vi "Write to TCP.vi"(8 "error in (no error)":errorcluster, 11 "Vessel in":refnum<class "Vessel.lvclass">) -> (0 "error out":errorcluster, 3 "Vessel out":refnum<class "Vessel.lvclass">)   [LabVIEW 2014, in "Vessel.lvclass"]
uses:
  Vessel.lvclass
  Vessel.lvclass/Vessel.ctl
  Library/Helping Routines/get_set_point (SubVI).vi
  Supervisor/Supervisor.lvclass
panel:
  out "Name":string
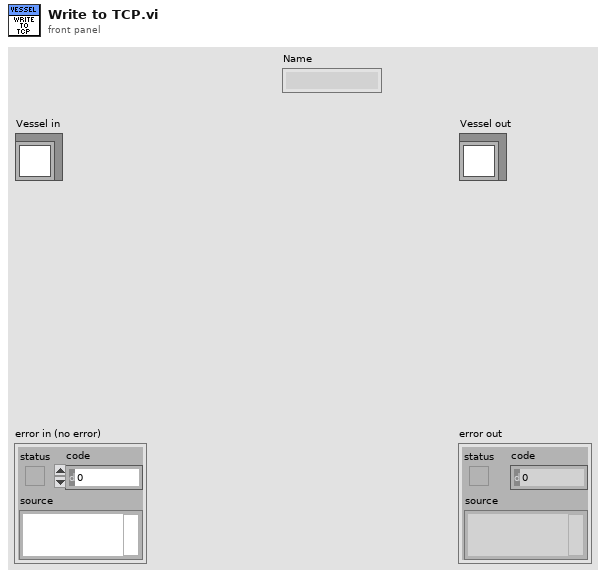
[diagram p1: front panel]
types:
  T1 = cluster{"Measured":cluster{"Eta":dbl[], "Nu":dbl[], "Eta Dot":dbl[], "Nu Dot":dbl[]}, "Estimated":cluster{"Eta":dbl[], "Nu":dbl[], "Eta Dot":dbl[], "Nu Dot":dbl[]}, "Desired":cluster{"Eta":dbl[], "Nu":dbl[], "Eta Dot":dbl[], "Nu Dot":dbl[]}, "Previous Desired":cluster{"Eta":dbl[], "Nu":dbl[], "Eta Dot":dbl[], "Nu Dot":dbl[]}, "tau":dbl[], "Altitude":cluster{"Measured":dbl, "Estimated":dbl, "Desired":dbl, "Previous Desired":dbl, "Approximated":dbl, "grad F":dbl[]}, "rpm":dbl[], "Attitude":cluster{"Theta Measured":dbl[], "Theta Estimated":dbl[], "Omega Measured":dbl[], "Omega Estimated":dbl[], "Gyro Bias":dbl[]}}
  T2 = cluster{"Set Origin":bool, "New WP":bool, "Types of Change":enum16{"Current NED", "Change NED"}, "Make Change":bool, "Optimal Heading":bool, "New SetPoint":cluster{"North":dbl, "East":dbl, "Depth":dbl, "Heading":dbl}, "Update Reference":cluster{"Mode Change":bool, "Current Position":dbl[]}, "Go":bool, "Go heading":bool}
  T3 = cluster{"Pressure +":bool, "Pressure -":bool, "Vacuum +":bool, "Vacuum -":bool}
  T4 = cluster{"In":bool, "Out":bool, "Rotate CW":bool, "Rotate CCW":bool}
  T5 = cluster{"Button 1":bool, "Button 2":bool, "Button 3":bool, "Button 4":bool, "Button 5":bool, "Button 6":bool, "Button 7":bool, "Button 8":bool, "Button 9":bool, "Button 10":bool, "Button 11":bool, "Button 12":bool, "POV Direction":i32}
  T6 = cluster{"Eta":dbl[], "Nu":dbl[], "Eta Dot":dbl[], "Nu Dot":dbl[]}
  T7 = cluster{"Theta Measured":dbl[], "Theta Estimated":dbl[], "Omega Measured":dbl[], "Omega Estimated":dbl[], "Gyro Bias":dbl[]}
  T8 = cluster{"Measured":dbl, "Estimated":dbl, "Desired":dbl, "Previous Desired":dbl, "Approximated":dbl, "grad F":dbl[]}
  T9 = cluster{"HPR":bool, "Sonar 1":bool, "Sonar 2":bool, "Doppler":bool, "Laser":bool, "KRAFT":bool, "Pan/Tilt":bool, "Transponder":bool, "Still Cam":bool, "HD Cam":bool, "UHI Cam":bool}
  T10 = cluster{"Power Switch":bool, "Upper Arm Up":bool, "Upper Arm Down":bool, "Lower Arm Up":bool, "Lower Arm Down":bool, "Arm Left":bool, "Arm Right":bool, "Claw Open":bool, "Claw Close":bool, "Rotate Clockwise":bool, "Rotate Counterclockwise":bool}
  T11 = cluster{"Light 1":bool, "Light 2":bool, "Light 3":bool, "Light 4":bool, "HMI 1":bool, "HMI 2":bool, "Light Intensity 1":i32, "Light Intensity 2":i32, "Light Intensity 3":i8}
  T12 = cluster{"Cam. No.":i32, "Cam Up":bool, "Cam Down":bool, "Cam Left":bool, "Cam Right":bool, "Zoom In":bool, "Zoom Out":bool, "Zoom In 2":bool, "Zoom Out 2":bool}
  T13 = cluster{"Altimeter Active":bool, "Beam select":i8, "Value":cluster{"Measured":dbl, "Estimated":dbl, "Desired":dbl, "Previous Desired":dbl, "Approximated":dbl}}
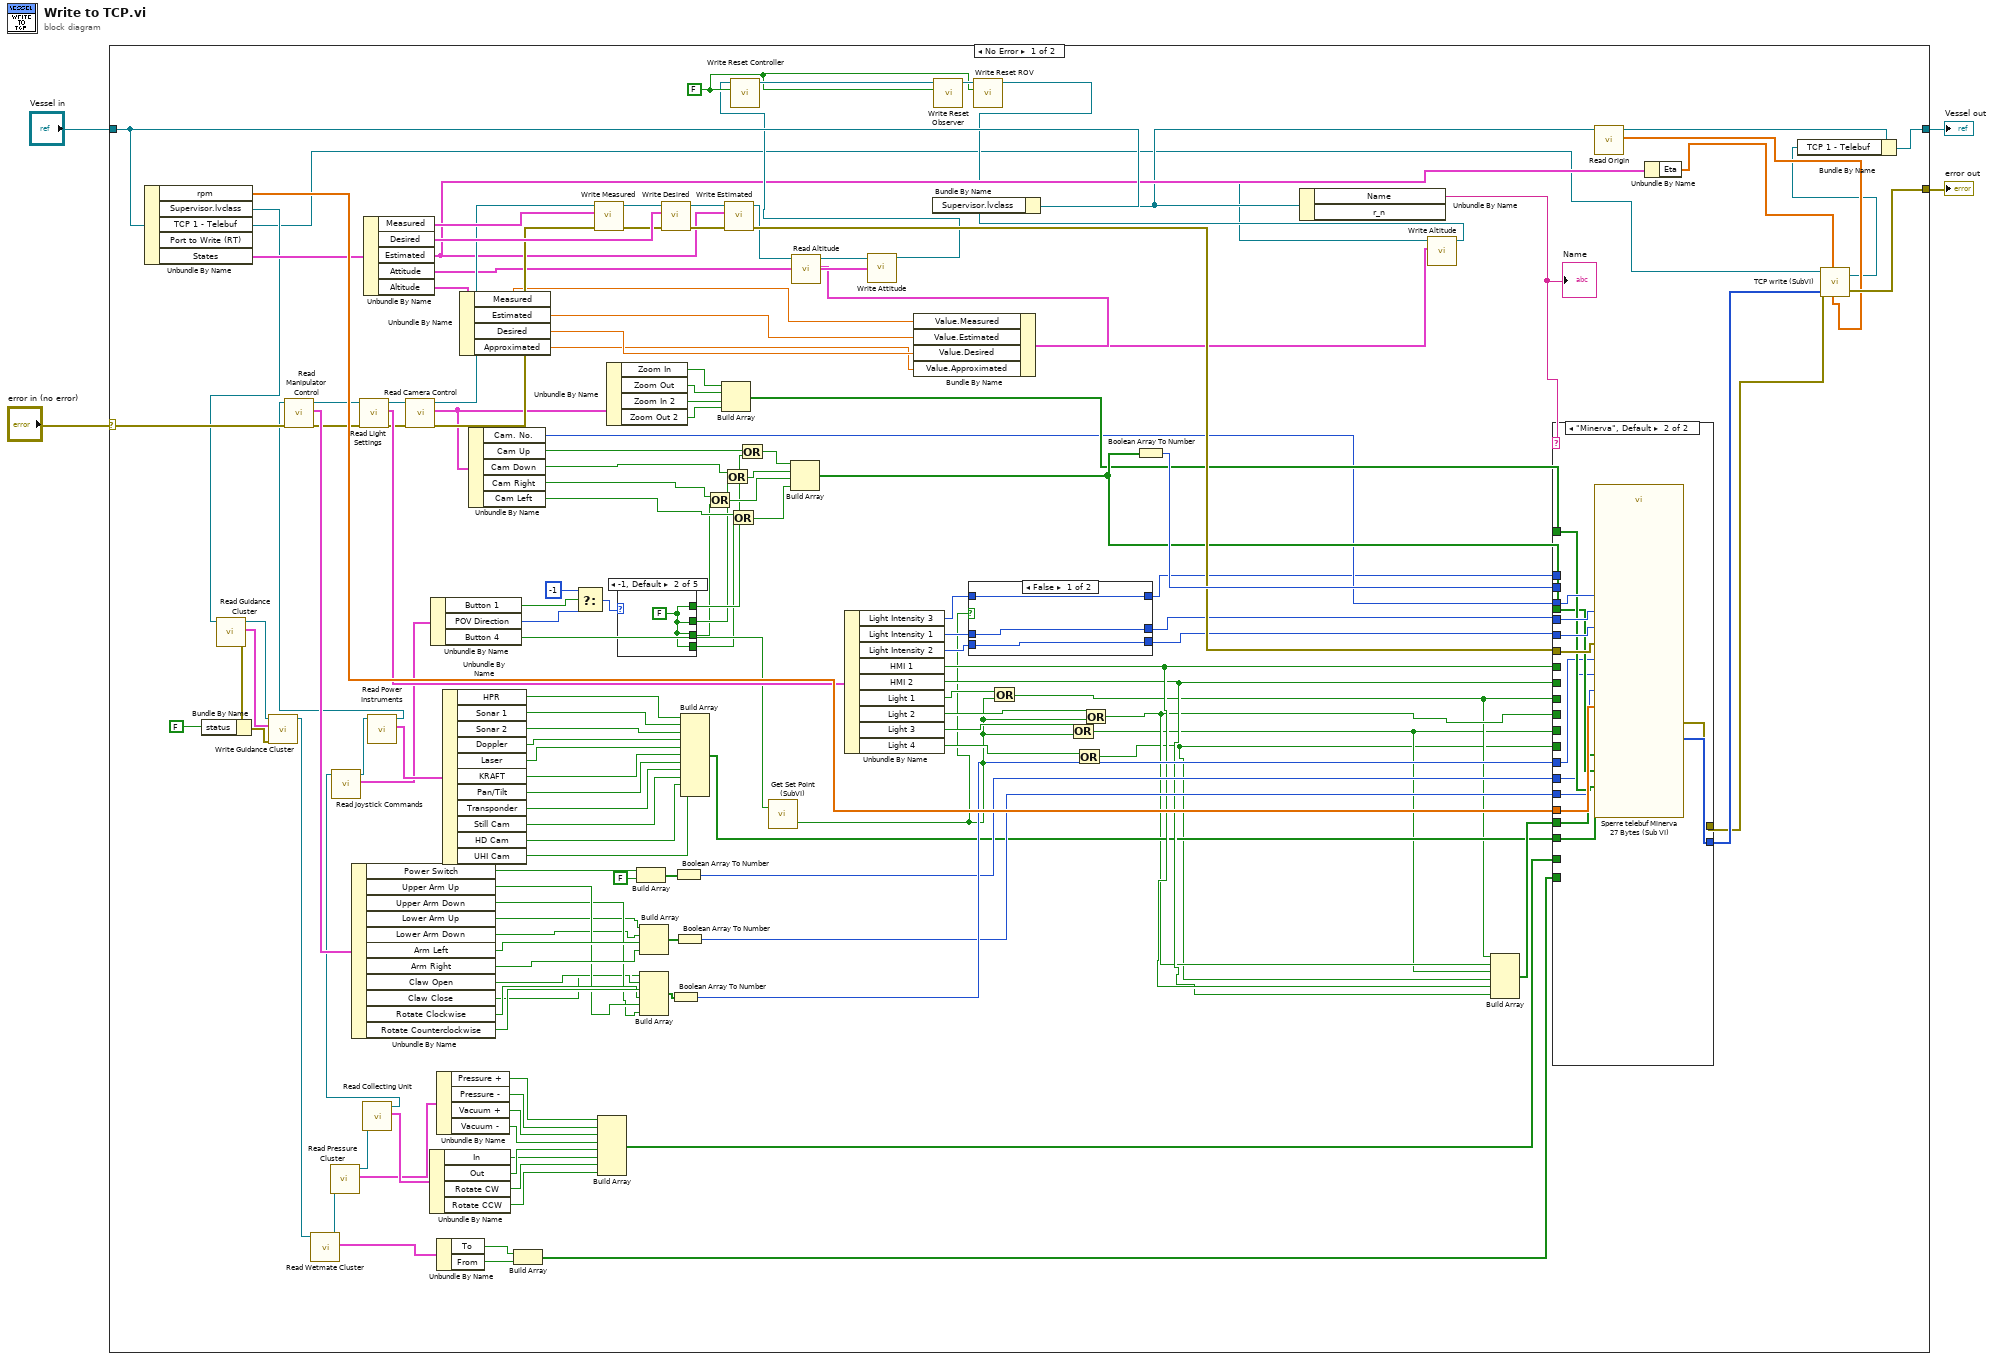
[diagram p0: block diagram]
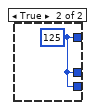
[diagram p2: hidden frame]
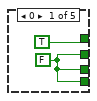
[diagram p3: hidden frame]
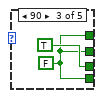
[diagram p4: hidden frame]
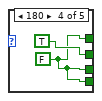
[diagram p5: hidden frame]
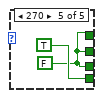
[diagram p6: hidden frame]
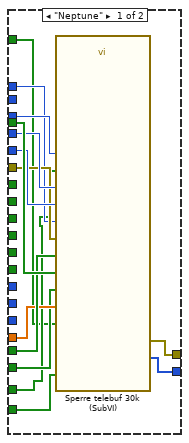
[diagram p7: hidden frame]
diagram:
  n1 = case shown="No Error" "error in (no error)" {
    selector: "error in (no error)" -> [w141 w197]
    tunnel: [w9 w197] -> w3
    tunnel: [w144 w196] -> w1
    tunnel: "Vessel in" -> [w133 w196]
    frame No Error {
      w121 = FALSE ("Reset Controller")
      n2 = Unbundle By Name(w133) -> ("rpm"=w154:dbl[], "Supervisor.lvclass"=w124:refnum<class "Supervisor.lvclass">, "TCP 1 - Telebuf"=w6:refnum<k5>, "States"=w138:T1)  [unwired: 1 out]
      n3 = call-dynamic "Read Guidance Cluster.vi"("Supervisor in"=w124) -> ("error out"=w126:errorcluster, "Guidance Cluster"=w65:T2, "Supervisor out"=w127:refnum<class "Supervisor.lvclass">)  [unwired: 8 in]
      n4 = Bundle By Name(cluster=w126, "status"=FALSE ("Set Origin")) -> (w66:errorcluster)
      n5 = call-dynamic "Write Guidance Cluster.vi"("error in (no error)"=w66, "Guidance Cluster"=w65, "Supervisor in"=w127) -> ("Supervisor out"=w73:refnum<class "Supervisor.lvclass">)  [unwired: 7 in, 1 out]
      n6 = call-dynamic "Read Wetmate Cluster.vi"("Supervisor in"=w73) -> ("Wetmate Cluster"=w71:cluster{"To":bool, "From":bool}, "Supervisor out"=w72:refnum<class "Supervisor.lvclass">)  [unwired: 8 in, 1 out]
      n7 = call-dynamic "Read Pressure Cluster.vi"("Supervisor in"=w72) -> ("Pressure Cluster"=w78:T3, "Supervisor out"=w79:refnum<class "Supervisor.lvclass">)  [unwired: 8 in, 1 out]
      n8 = call-dynamic "Read Collecting Unit.vi"("Supervisor in"=w79) -> ("Collecting Unit"=w103:T4, "Supervisor out"=w63:refnum<class "Supervisor.lvclass">)  [unwired: 8 in, 1 out]
      n9 = call-dynamic "Read Joystick Commands.vi"("Supervisor in"=w63) -> ("Joystick Commands"=w61:T5, "Supervisor out"=w62:refnum<class "Supervisor.lvclass">)  [unwired: 8 in, 1 out]
      n10 = Unbundle By Name(w138) -> ("Measured"=w137:T6, "Desired"=w136:T6, "Estimated"=w67:T6, "Attitude"=w92:T7, "Altitude"=w85:T8)
      n11 = call-dynamic "Read Power Instruments.vi"("Supervisor in"=w62) -> ("Power Instruments"=w115:T9, "Supervisor out"=w116:refnum<class "Supervisor.lvclass">)  [unwired: 8 in, 1 out]
      n12 = call-dynamic "Read Manipulator Control.vi"("error in (no error)"=w141, "Supervisor in"=w116) -> ("error out"=w140:errorcluster, "Manipulator Control"=w151:T10, "Supervisor out"=w143:refnum<class "Supervisor.lvclass">)  [unwired: 7 in]
      n13 = Unbundle By Name(w151) -> ("Power Switch"=w150:bool, "Upper Arm Up"=w29:bool, "Upper Arm Down"=w28:bool, "Lower Arm Up"=w27:bool, "Lower Arm Down"=w26:bool, "Arm Left"=w34:bool, "Arm Right"=w33:bool, "Claw Open"=w25:bool, "Claw Close"=w24:bool, "Rotate Clockwise"=w30:bool, "Rotate Counterclockwise"=w31:bool)
      n14 = call-dynamic "Read Light Settings.vi"("error in (no error)"=w140, "Supervisor in"=w143) -> ("error out"=w139:errorcluster, "Light Settings"=w152:T11, "Supervisor out"=w142:refnum<class "Supervisor.lvclass">)  [unwired: 7 in]
      n15 = call-dynamic "Read Camera Control.vi"("error in (no error)"=w139, "Supervisor in"=w142) -> ("error out"=w132:errorcluster, "Camera Control"=w97:T12, "Supervisor out"=w134:refnum<class "Supervisor.lvclass">)  [unwired: 7 in]
      n16 = Unbundle By Name(w103) -> ("In"=w101:bool, "Out"=w102:bool, "Rotate CW"=w100:bool, "Rotate CCW"=w99:bool)
      n17 = Unbundle By Name(w61) -> ("Button 1"=w39:bool, "POV Direction"=w38:i32, "Button 4"=w60:bool)
      n18 = Unbundle By Name(w78) -> ("Pressure +"=w77:bool, "Pressure -"=w76:bool, "Vacuum +"=w75:bool, "Vacuum -"=w74:bool)
      n19 = Unbundle By Name(w71) -> ("To"=w70:bool, "From"=w69:bool)
      n20 = Unbundle By Name(w115) -> ("HPR"=w114:bool, "Sonar 1"=w113:bool, "Sonar 2"=w112:bool, "Doppler"=w111:bool, "Laser"=w110:bool, "KRAFT"=w109:bool, "Pan/Tilt"=w108:bool, "Transponder"=w107:bool, "Still Cam"=w106:bool, "HD Cam"=w105:bool, "UHI Cam"=w12:bool)
      n21 = Unbundle By Name(w85) -> ("Measured"=w84:dbl, "Estimated"=w83:dbl, "Desired"=w82:dbl, "Approximated"=w80:dbl)
      n22 = Unbundle By Name(w97) -> ("Cam. No."=w64:i32, "Cam Up"=w51:bool, "Cam Down"=w49:bool, "Cam Right"=w47:bool, "Cam Left"=w45:bool)
      n23 = Build Array(w70, w69) -> (w68:bool[])
      n24 = Select(t=-1, s=w39, f=w38) -> (s? t:f=w37:i32)
      n25 = call-dynamic "Write Measured.vi"("error in (no error)"=w132, "Measured"=w137, "Supervisor in"=w134) -> ("error out"=w131:errorcluster, "Supervisor out"=w135:refnum<class "Supervisor.lvclass">)  [unwired: 7 in]
      n26 = Build Array(w77, w76, w75, w74, w102, w101, w100, w99) -> (w98:bool[])
      n27 = Unbundle By Name(w97) -> ("Zoom In"=w96:bool, "Zoom Out"=w95:bool, "Zoom In 2"=w94:bool, "Zoom Out 2"=w93:bool)
      n28 = case shown="-1, Default" w37 {
        tunnel: [TRUE w161 w162 w164 w166] -> w43
        tunnel: [w159 w161 w162 TRUE w166] -> w42
        tunnel: [w159 w161 TRUE w164 w166] -> w41
        tunnel: [w159 w161 w162 w164 TRUE] -> w40
        frame 0 {
          w159 = FALSE
        }
        frame -1, Default {
          w161 = FALSE
        }
        frame 90 {
          w162 = FALSE
        }
        frame 180 {
          w164 = FALSE
        }
        frame 270 {
          w166 = FALSE
        }
      }
      n29 = Build Array(w150, FALSE ("element")) -> (w149:bool[])
      n30 = Build Array(w27, w26, w34, w33) -> (w32:bool[])
      n31 = Build Array(w24, w25, w31, w30, w29, w28) -> (w148:bool[])
      n32 = call-dynamic "Write Desired.vi"("error in (no error)"=w131, "Desired"=w136, "Supervisor in"=w135) -> ("error out"=w129:errorcluster, "Supervisor out"=w130:refnum<class "Supervisor.lvclass">)  [unwired: 7 in]
      n33 = Boolean Array To Number(Boolean array=w148) -> (number=w147:u32)
      n34 = Boolean Array To Number(Boolean array=w149) -> (number=w146:u32)
      n35 = Boolean Array To Number(Boolean array=w32) -> (number=w145:u32)
      n36 = Build Array(w114, w113, w112, w111, w110, w109, w108, w107, w106, w105, w12) -> (w104:bool[])
      n37 = Or(x=w47, y=w41) -> (x .or. y?=w46:bool)
      n38 = Build Array(w96, w95, w94, w93) -> (w81:bool[])
      n39 = Or(x=w49, y=w42) -> (x .or. y?=w48:bool)
      n40 = call-dynamic "Write Estimated.vi"("error in (no error)"=w129, "Estimated"=w67, "Supervisor in"=w130) -> ("error out"=w128:errorcluster, "Supervisor out"=w89:refnum<class "Supervisor.lvclass">)  [unwired: 7 in]
      n41 = Or(x=w45, y=w40) -> (x .or. y?=w44:bool)
      n42 = Or(x=w51, y=w43) -> (x .or. y?=w50:bool)
      n43 = call-poly "Get Set Point (SubVI).vi"("auto set  in"=w60) -> ("auto set"=w13:bool)  [unwired: 1 in, 1 out]
      n44 = Build Array(w50, w48, w46, w44) -> (w120:bool[])
      n45 = call-dynamic "Read Altitude.vi"("Supervisor in"=w89) -> ("Altitude"=w90:T13, "Supervisor out"=w88:refnum<class "Supervisor.lvclass">)  [unwired: 8 in, 1 out]
      n46 = Unbundle By Name(w152) -> ("Light Intensity 3"=w18:i8, "Light Intensity 1"=w16:i32, "Light Intensity 2"=w14:i32, "HMI 1"=w119:bool, "HMI 2"=w118:bool, "Light 1"=w59:bool, "Light 2"=w58:bool, "Light 3"=w55:bool, "Light 4"=w53:bool)
      n47 = call-dynamic "Write Attitude.vi"("Attitude"=w92, "Supervisor in"=w88) -> ("Supervisor out"=w91:refnum<class "Supervisor.lvclass">)  [unwired: 8 in, 1 out]
      n48 = call-dynamic "Write Reset Controller.vi"("Reset Controller"=w121, "Supervisor in"=w91) -> ("Supervisor out"=w123:refnum<class "Supervisor.lvclass">)  [unwired: 8 in, 1 out]
      n49 = Bundle By Name(cluster=w90, "Value.Measured"=w84, "Value.Estimated"=w83, "Value.Desired"=w82, "Value.Approximated"=w80) -> (w87:T13)
      n50 = call-dynamic "Write Reset Observer.vi"("Reset Observer"=w121, "Supervisor in"=w123) -> ("Supervisor out"=w122:refnum<class "Supervisor.lvclass">)  [unwired: 8 in, 1 out]
      n51 = case shown="False" w13 {
        tunnel: [w157 w158] -> w19
        tunnel: w18 -> [w157 _]
        tunnel: [w156 w158] -> w17
        tunnel: w16 -> [w156 _]
        tunnel: [w155 w158] -> w15
        tunnel: w14 -> [w155 _]
        frame False {
        }
        frame True {
          w158 = i8 125 ("Light Intensity 3")
        }
      }
      n52 = call-dynamic "Write Reset ROV.vi"("Reset ROV"=w121, "Supervisor in"=w122) -> ("Supervisor out"=w21:refnum<class "Supervisor.lvclass">)  [unwired: 8 in, 1 out]
      n53 = Or(x=w59, y=w13) -> (x .or. y?=w56:bool)
      n54 = Or(x=w55, y=w13) -> (x .or. y?=w54:bool)
      n55 = Or(x=w53, y=w13) -> (x .or. y?=w52:bool)
      n56 = Or(x=w58, y=w13) -> (x .or. y?=w57:bool)
      n57 = Boolean Array To Number(Boolean array=w120) -> (number=w153:u32)
      n58 = call-dynamic "Write Altitude.vi"("Altitude"=w87, "Supervisor in"=w21) -> ("Supervisor out"=w86:refnum<class "Supervisor.lvclass">)  [unwired: 8 in, 1 out]
      n59 = Bundle By Name(cluster=w133, "Supervisor.lvclass"=w86) -> (w23:refnum<class "Vessel.lvclass">)
      n60 = Unbundle By Name(w23) -> ("Name"=w20:string)  [unwired: 1 out]
      "Name" <- w20
      n61 = Build Array(w56, w57, w54, w52, w119, w118) -> (w117:bool[])
      n62 = case shown="\"Minerva\", Default" w20 {
        tunnel: w154 -> [w173 w190]
        tunnel: [w181 w194] -> w10
        tunnel: [w180 w193] -> w5
        tunnel: w119 -> [_ _]
        tunnel: w118 -> [_ _]
        tunnel: w56 -> [_ _]
        tunnel: w57 -> [_ _]
        tunnel: w54 -> [_ _]
        tunnel: w52 -> [_ _]
        tunnel: w17 -> [w177 w192]
        tunnel: w15 -> [w176 w191]
        tunnel: w153 -> [_ _]
        tunnel: w64 -> [w175 w195]
        tunnel: w147 -> [_ w185]
        tunnel: w146 -> [_ w184]
        tunnel: w145 -> [_ w183]
        tunnel: w128 -> [w174 w188]
        tunnel: w120 -> [w179 w186]
        tunnel: w117 -> [w178 w189]
        tunnel: w104 -> [w172 w182]
        tunnel: w19 -> [w171 _]
        tunnel: w98 -> [w170 _]
        tunnel: w81 -> [w169 w187]
        tunnel: w68 -> [w168 _]
        frame "Neptune" {
          n63 = call "Sperre telebuf 30k (SubVI).vi"("Thruster rpms"=w173, "pan tilt"=w179, "Lights/HMI"=w178, "Wetmate"=w168, "error in"=w174, "dim 1"=w177, "Power Instruments"=w172, "dim 2"=w176, "Collecting Unit"=w170, "dim 34"=w171, "Zoom 1-2"=w169, "cam no"=w175) -> ("telebuf out"=w181:u8[], "error IO"=w180:errorcluster)  [unwired: 6 in]
        }
        frame "Minerva", Default {
          n64 = call "Sperre telebuf Minerva 27 Bytes (Sub VI).vi"("Thruster rpms"=w190, "manip1"=w185, "manip2"=w184, "manip3"=w183, "Pan_tilt"=w186, "error in"=w188, "dim 1+2"=w192, "Lights_HMI"=w189, "dim 3+4"=w191, "Zoom"=w187, "Power"=w182, "camera"=w195) -> ("telebuf"=w194:u8[], "error IO"=w193:errorcluster)  [unwired: 6 in]
        }
      }
      n65 = call-dynamic "Read Origin.vi"("Vessel in"=w23) -> ("Origin"=w8:dbl[], "Vessel out"=w22:refnum<class "Vessel.lvclass">)  [unwired: 8 in, 1 out]
      n66 = Unbundle By Name(w67) -> ("Eta"=w11:dbl[])
      n67 = call "TCP write (SubVI).vi"("States"=w8, "CO_NED"=w11, "error IO"=w5, "Array"=w10, "TCP Network Connection Refnum In"=w6) -> ("error out"=w9:errorcluster, "TCP Network Connection Refnum Out"=w7:refnum<k5>)  [unwired: 1 in]
      n68 = Bundle By Name(cluster=w22, "TCP 1 - Telebuf"=w7) -> (w144:refnum<class "Vessel.lvclass">)
    }
    frame Error {
    }
  }
  "error out" <- w3
  "Vessel out" <- w1
